vi "Analog_Input_16Channels_W24I5.vi"(1 "IO":T1={"AI 0"="Mod2/AI0", "AI 1"="Mod2/AI0", "AI 2"="Mod2/AI0", "AI 3"="Mod2/AI0", "AI 4"="Mod2/AI0", "AI 5"="Mod2/AI0", "AI 6"="Mod2/AI0", "AI 7"="Mod2/AI0", "AI 8"="Mod2/AI0", "AI 9"="Mod2/AI0", "AI 10"="Mod2/AI0", "AI 11"="Mod2/AI0", "AI 12"="Mod2/AI0", "AI 13"="Mod2/AI0", "AI 14"="Mod2/AI0", "AI 15"="Mod2/AI0"}) -> (0 "Values":fxp<+/-,24,5>[](array[numeric]))   [LabVIEW 2019, in "FPGA Wizard Templates.lvlib"]
uses:
  FPGA Wizard Templates.lvlib
  <vilib>/eio/EIONode/EIONode.xnode
  <vilib>/rvi/eio/common/nirviEmuTemplateMethod_errors.vi
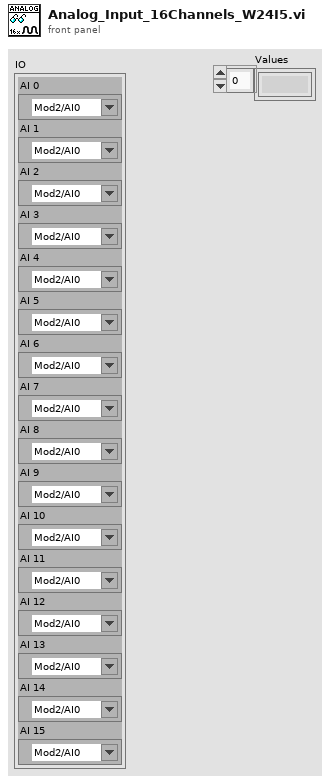
[diagram p1: front panel]
types:
  T1 = cluster{"AI 0":refnum<k21>, "AI 1":refnum<k21>, "AI 2":refnum<k21>, "AI 3":refnum<k21>, "AI 4":refnum<k21>, "AI 5":refnum<k21>, "AI 6":refnum<k21>, "AI 7":refnum<k21>, "AI 8":refnum<k21>, "AI 9":refnum<k21>, "AI 10":refnum<k21>, "AI 11":refnum<k21>, "AI 12":refnum<k21>, "AI 13":refnum<k21>, "AI 14":refnum<k21>, "AI 15":refnum<k21>}
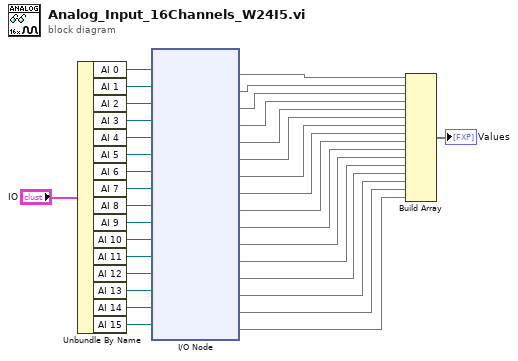
[diagram p0: block diagram]
diagram:
  n1 = Unbundle By Name("IO") -> ("AI 0"=w33:refnum<k21>, "AI 1"=w32:refnum<k21>, "AI 2"=w31:refnum<k21>, "AI 3"=w30:refnum<k21>, "AI 4"=w29:refnum<k21>, "AI 5"=w28:refnum<k21>, "AI 6"=w27:refnum<k21>, "AI 7"=w26:refnum<k21>, "AI 8"=w17:refnum<k21>, "AI 9"=w16:refnum<k21>, "AI 10"=w15:refnum<k21>, "AI 11"=w14:refnum<k21>, "AI 12"=w13:refnum<k21>, "AI 13"=w12:refnum<k21>, "AI 14"=w11:refnum<k21>, "AI 15"=w10:refnum<k21>)
  n2 = xnode "I/O Node"("FPGA I/O In"=w33, "FPGA I/O In"=w32, "FPGA I/O In"=w31, "FPGA I/O In"=w30, "FPGA I/O In"=w29, "FPGA I/O In"=w28, "FPGA I/O In"=w27, "FPGA I/O In"=w26, "FPGA I/O In"=w17, "FPGA I/O In"=w16, "FPGA I/O In"=w15, "FPGA I/O In"=w14, "FPGA I/O In"=w13, "FPGA I/O In"=w12, "FPGA I/O In"=w11, "FPGA I/O In"=w10) -> ("I/O Item"=w25, "I/O Item"=w24, "I/O Item"=w23, "I/O Item"=w22, "I/O Item"=w21, "I/O Item"=w20, "I/O Item"=w19, "I/O Item"=w18, "I/O Item"=w9, "I/O Item"=w8, "I/O Item"=w7, "I/O Item"=w6, "I/O Item"=w5, "I/O Item"=w4, "I/O Item"=w3, "I/O Item"=w2)  [unwired: 16 out]
  n3 = Build Array(w25, w24, w23, w22, w21, w20, w19, w18, w9, w8, w7, w6, w5, w4, w3, w2) -> (→"Values":void[])
